vi "reflect_and_rotate_point.vi"(9 "Point":cluster{"X":sgl, "Y":sgl} {"Y" format="%.2f"; "X" format="%.2f"}, 10 "reflect about the x axis?":bool, 11 "rotation angle (radians)":sgl) -> (1 "transformed point":cluster{"X":sgl, "Y":sgl} {"Y" format="%.2f"; "X" format="%.2f"})   [LabVIEW 2019]
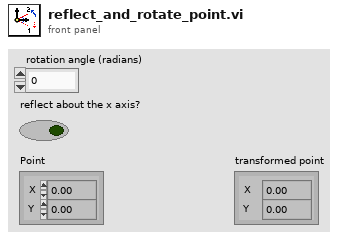
[diagram p1: front panel]
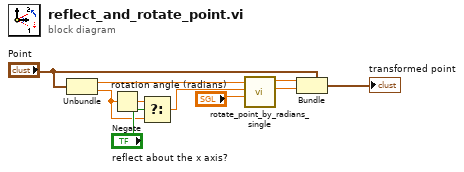
[diagram p0: block diagram]
diagram:
  n1 = Unbundle("Point") -> ("X"=w2:sgl, "Y"=w5:sgl)
  n2 = Negate(x=w5) -> (-x=w10:sgl)
  n3 = Select(t=w10, s="reflect about the x axis?", f=w5) -> (s? t:f=w1:sgl)
  n4 = call "rotate_point_by_radians_single.vi"("theta"="rotation angle (radians)", "y"=w1, "x"=w2) -> ("y out"=w3:sgl, "x out"=w4:sgl)  [unwired: 7 in]
  n5 = Bundle(cluster="Point", "X"=w4, "Y"=w3) -> (→"transformed point":cluster{"X":sgl, "Y":sgl})
